vi "AbbreviateModifications.vi"(4 "svnString":string) -> (1 "VInames":string)   [LabVIEW 2022 SP3]
uses:
  <vilib>/Utility/error.llb/Trim Whitespace One-Sided.vi
  <vilib>/regexp/Match Regular Expression.xnode
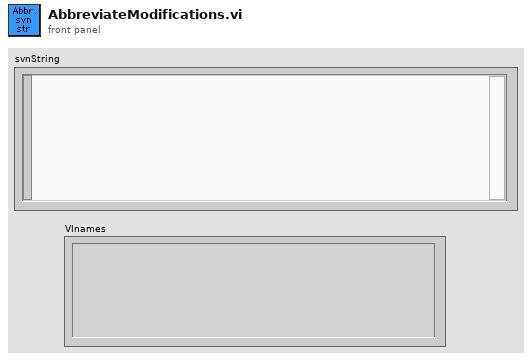
[diagram p1: front panel]
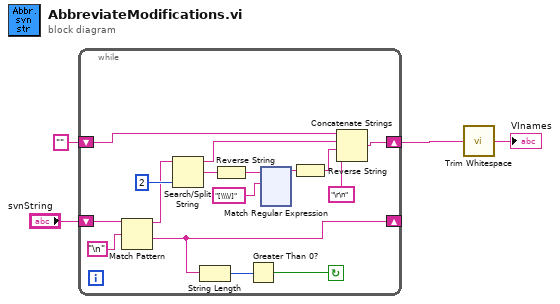
[diagram p0: block diagram]
diagram:
  n1 = while {
    shift-right: [w17] -> _
    shift-left: "svnString" -> [w20]
    shift-right: [w18] -> w2
    shift-left: "" -> [w19]
    stop <- w15 continue-if-true
    n2 = Match Pattern(string=w20, regular expression="\n") -> (before substring=w9:string, after substring=w17:string)  [unwired: 1 in, 2 out]
    n3 = Search/Split String(string=w9, offset (0)=2) -> (substring before match=w13:string, match + rest of string=w6:string)  [unwired: 1 in, 1 out]
    n4 = String Length(string=w17) -> (length=w16:i32)
    n5 = Reverse String(1:w6) -> (0:w8:string)
    n6 = Greater Than 0?(x=w16) -> (x > 0?=w15:bool)
    n7 = xnode "Match Regular Expression"("input string"=w8, "regular expression"="[\\\\/]") -> ("before match"=w10:string)  [unwired: 4 in, 4 out]
    n8 = Reverse String(1:w10) -> (0:w5:string)
    n9 = Concatenate Strings(w19, w13, w5, "\r\n" ("regular expression")) -> (w18:string)
  }
  n10 = call <vilib>:"Trim Whitespace.vi"("string"=w2) -> ("trimmed string"=→"VInames":string)  [unwired: 1 in]
